vi "Read_Output.vi"(8 "error in (no error)":errorcluster caption="entrée d'erreur (pas d'erreur)", 11 "Class Power_Supply Rigol DP800 en entrée":refnum<class "Class Power_Supply Rigol DP800.lvclass">) -> (0 "error out":errorcluster caption="sortie d'erreur", 3 "Class Power_Supply Rigol DP800 en sortie":refnum<class "Class Power_Supply Rigol DP800.lvclass">)   [LabVIEW 2020, in "Library Instrument & Equipement.lvlib" / "Library Power_Supply.lvlib" / "Class Power_Supply Rigol DP800.lvclass"]
uses:
  Class Power_Supply Rigol DP800.lvclass
  C:/Users/ngarcin/OneDrive - Altyor/Standard TB/Class/Power_Supply/Power_Supply (Default)/Power_Supply (Default).lvclass
  Class Power_Supply Rigol DP800.lvclass/Class Power_Supply Rigol DP800.ctl
  RIGOL DP800 Series/RIGOL DP800 Series.lvlib
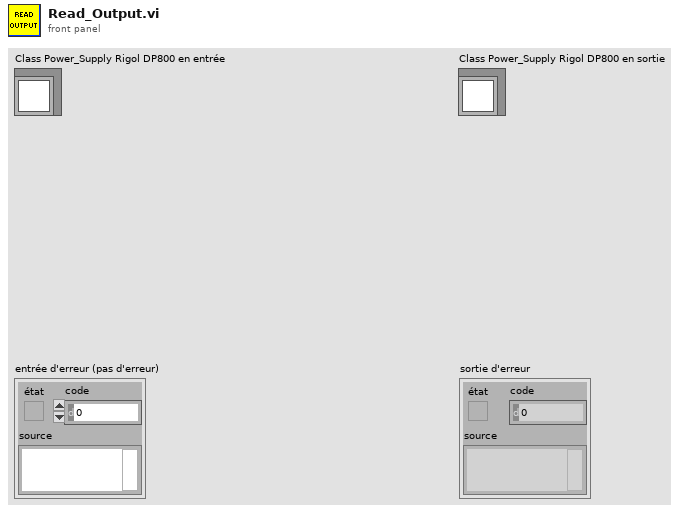
[diagram p1: front panel]
types:
  T1 = cluster{"Power":dbl, "Voltage":dbl, "Current":dbl}
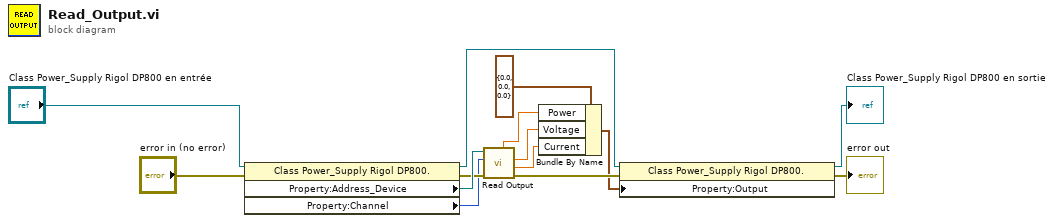
[diagram p0: block diagram]
diagram:
  n1 = property class="Class Power_Supply Rigol DP800."(reference="Class Power_Supply Rigol DP800 en entrée", error in="error in (no error)") -> (reference out=w11:refnum<class "Class Power_Supply Rigol DP800.lvclass">, error out=w10:errorcluster, "Property:Address_Device"=w13:refnum<visa-resource-name>, "Property:Channel"=w8:i32)
  n2 = call "Read Output.vi"("error in (no error)"=w10, "Channel (0: 30V Channel)"=w8, "VISA resource name"=w13) -> ("error out"=w9:errorcluster, "Actual Current Level (A)"=w4:dbl, "Actual Voltage Level (V)"=w5:dbl, "Actual Power Level (W)"=w6:dbl)  [unwired: 4 in, 1 out]
  n3 = Bundle By Name(cluster=T1 {"Power"=0.0, "Voltage"=0.0, "Current"=0.0} ("Output"), "Power"=w6, "Voltage"=w5, "Current"=w4) -> (w3:T1)
  n4 = property class="Class Power_Supply Rigol DP800."(reference=w11, error in=w9, "Property:Output"=w3) -> (reference out=→"Class Power_Supply Rigol DP800 en sortie":refnum<class "Class Power_Supply Rigol DP800.lvclass">, error out=→"error out":errorcluster)
